vi "HP53220 Measure Frequency w Waveform.vi"(0 "Channel(1,2,3)":enum16{"Channel 1", "Channel 2", "Channel 3"}(ring), 1 "Gate Time":dbl=1.0 min=0.0 max=1000.0 step=0.1 format="%.2f", 5 "Number of Readings":i32=1 min=1, 7 "GPIB Bus":i32 min=0 max=5, 9 "GPIB Address":i16=3 max=31, 11 "error in":errorcluster) -> (2 "Symmetry":dbl format="%.6f", 3 "Frequency":dbl format="%.6f", 4 "Vmax":dbl format="%.6f", 6 "Vmin":dbl format="%.6f", 8 "RTime":dbl format="%.6f", 10 "FTime":dbl format="%.6f", 15 "error out":errorcluster)   [LabVIEW 2023]
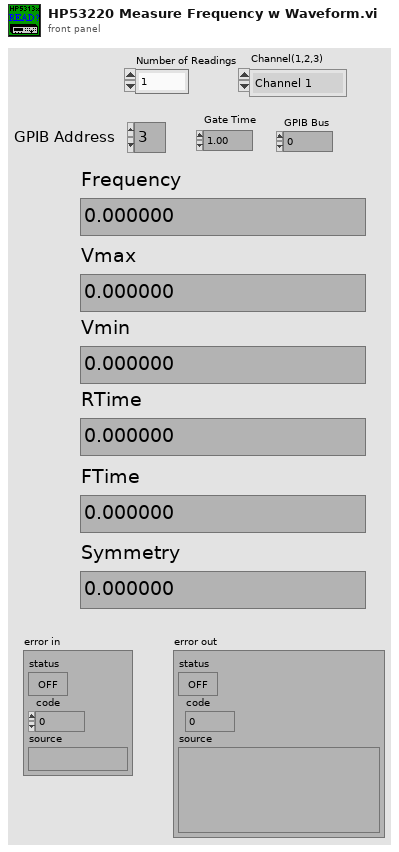
[diagram p1: front panel]
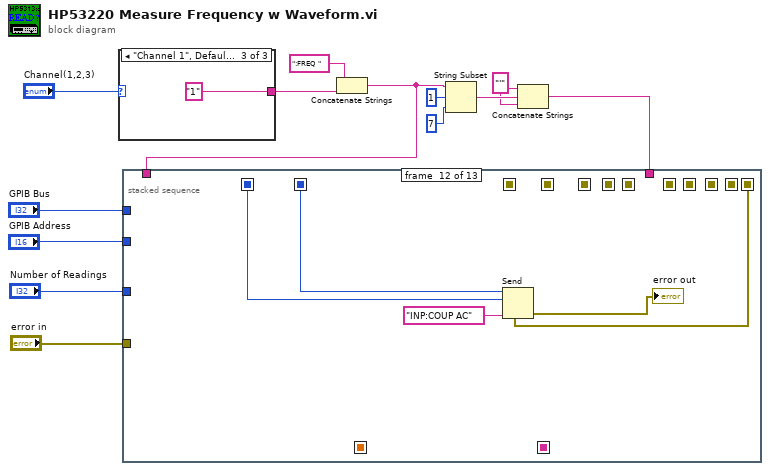
[diagram p0: block diagram]
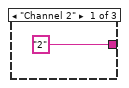
[diagram p2: hidden frame]
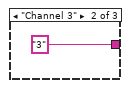
[diagram p3: hidden frame]
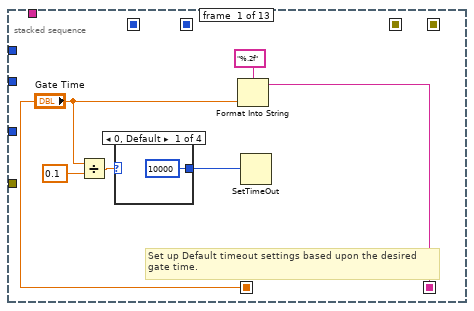
[diagram p4: hidden frame]
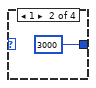
[diagram p5: hidden frame]
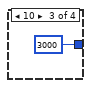
[diagram p6: hidden frame]
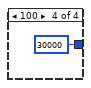
[diagram p7: hidden frame]
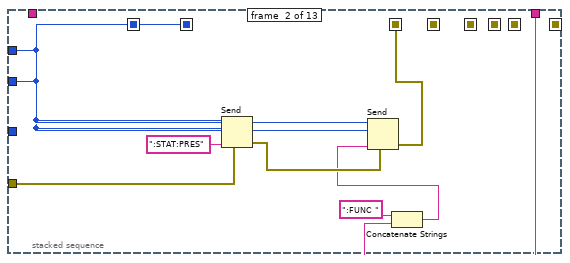
[diagram p8: hidden frame]
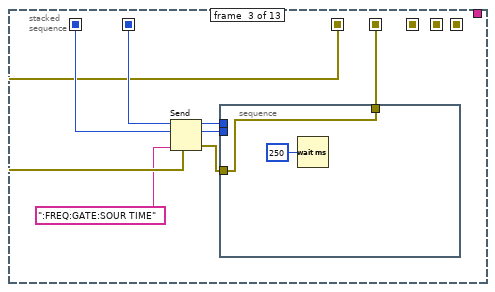
[diagram p9: hidden frame]
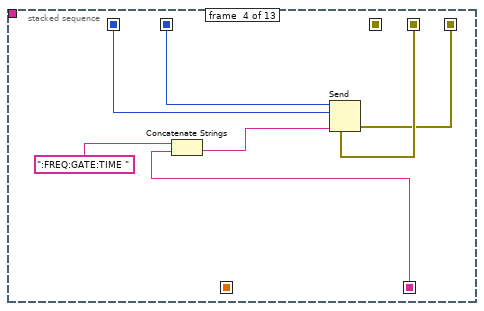
[diagram p10: hidden frame]
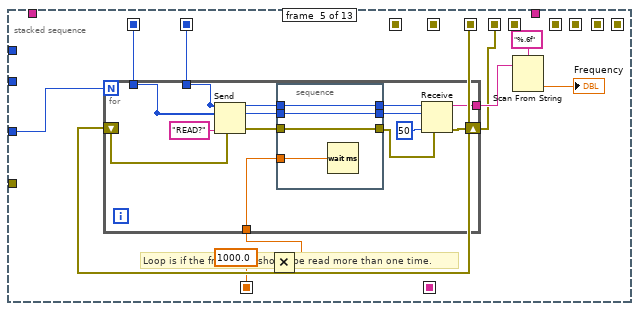
[diagram p11: hidden frame]
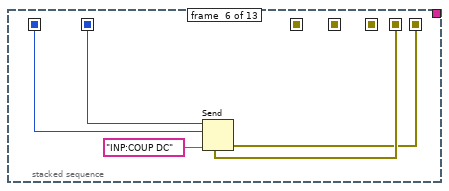
[diagram p12: hidden frame]
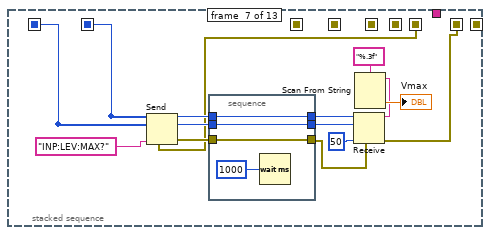
[diagram p13: hidden frame]
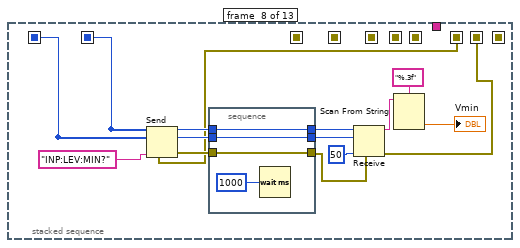
[diagram p14: hidden frame]
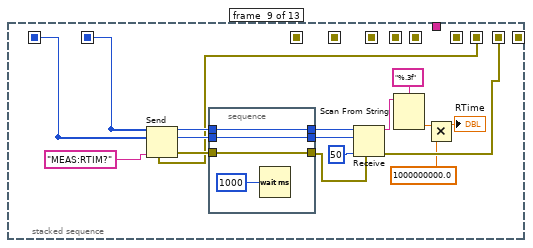
[diagram p15: hidden frame]
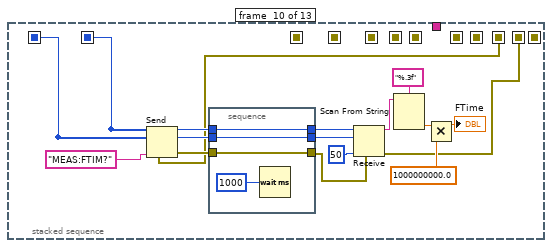
[diagram p16: hidden frame]
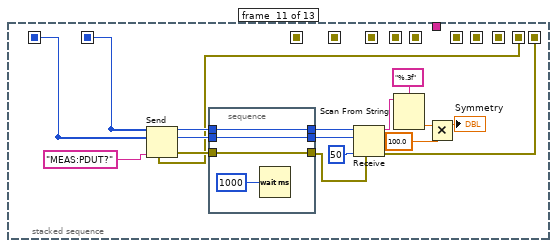
[diagram p17: hidden frame]
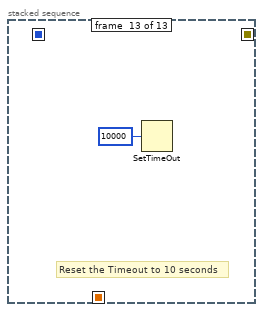
[diagram p18: hidden frame]
diagram:
  w4 = "'"
  n1 = case shown="\"Channel 1\", Default" "Channel(1,2,3)" {
    tunnel: ["2" "3" "1"] -> w10
    frame "Channel 2" {
    }
    frame "Channel 3" {
    }
    frame "Channel 1", Default {
    }
  }
  n2 = Concatenate Strings(":FREQ ", w10) -> (w8:string)
  n3 = String Subset(string=w8, offset (0)=1, length (rest)=7 ("length (rest)")) -> (substring=w5:string)
  n4 = Concatenate Strings(w4, w5, w4) -> (w3:string)
  n5 = stacked-sequence {
    seq-local: [_ w28 _ _ _ _ _ _ _ _ _ _ _] -> [_ _ w40 w50 w55 w81 w89 w106 w125 w144 w163 w177 _]
    seq-local: [w21 _ _ _ _ _ _ _ _ _ _ _ _] -> [_ _ _ w48 _ _ _ _ _ _ _ _ _]
    seq-local: [_ w29 _ _ _ _ _ _ _ _ _ _ _] -> [_ _ w41 w47 w56 w82 w90 w107 w126 w145 w164 w176 _]
    seq-local: [_ w34 _ _ _ _ _ _ _ _ _ _ _] -> [_ _ w39 _ _ _ _ _ _ _ _ _ _]
    seq-local: [_ _ w37 _ _ _ _ _ _ _ _ _ _] -> [_ _ _ w46 _ _ _ _ _ _ _ _ _]
    seq-local: [_ _ _ w45 _ _ _ _ _ _ _ _ _] -> [_ _ _ _ w58 _ _ _ _ _ _ _ _]
    seq-local: ["Gate Time" _ _ _ _ _ _ _ _ _ _ _ _] -> [_ _ _ _ w54 _ _ _ _ _ _ _ _]
    seq-local: [_ _ _ _ w51 _ _ _ _ _ _ _ _] -> [_ _ _ _ _ w79 _ _ _ _ _ _ _]
    seq-local: [_ _ _ _ _ w78 _ _ _ _ _ _ _] -> [_ _ _ _ _ _ w88 _ _ _ _ _ _]
    seq-local: [_ _ _ _ _ _ w83 _ _ _ _ _ _] -> [_ _ _ _ _ _ _ w101 _ _ _ _ _]
    seq-local: [_ _ _ _ _ _ _ w100 _ _ _ _ _] -> [_ _ _ _ _ _ _ _ w121 _ _ _ _]
    seq-local: [_ _ _ _ _ _ _ _ w120 _ _ _ _] -> [_ _ _ _ _ _ _ _ _ w137 _ _ _]
    seq-local: [_ _ _ _ _ _ _ _ _ w136 _ _ _] -> [_ _ _ _ _ _ _ _ _ _ w159 _ _]
    seq-local: [_ _ _ _ _ _ _ _ _ _ w158 _ _] -> [_ _ _ _ _ _ _ _ _ _ _ w175 _]
    tunnel: "GPIB Address" -> [_ w28 _ _ _ _ _ _ _ _ _ _ _]
    tunnel: "GPIB Bus" -> [_ w29 _ _ _ _ _ _ _ _ _ _ _]
    tunnel: w8 -> [_ _ _ _ _ _ _ _ _ _ _ _ _]
    tunnel: w3 -> [_ w30 _ _ _ _ _ _ _ _ _ _ _]
    tunnel: "error in" -> [_ w27 _ _ _ _ _ _ _ _ _ _ _]
    tunnel: "Number of Readings" -> [_ _ _ _ w57 _ _ _ _ _ _ _ _]
    frame #0 {
      # "Set up Default timeout settings based upon the desired \ngate time."
      n6 = Divide(x="Gate Time", y=0.1) -> (x/y=w19:dbl)
      n7 = case shown="0, Default" w19 {
        tunnel: [10000 3000 3000 30000] -> w20
        frame 0, Default {
        }
        frame 1 {
        }
        frame 10 {
        }
        frame 100 {
        }
      }
      n8 = Format Into String(format string="%.2f" ("Format String"), "Gate Time") -> (resulting string=w21:string)  [unwired: 2 in, 1 out]
      n9 = SetTimeOut(1:w20) -> ()  [unwired: 1 out]
    }
    frame #1 {
      n10 = Send(0:w29, 2:w28, 4:w27, 5:":STAT:PRES" ("data string")) -> (8:w33:errorcluster)  [unwired: 1 in, 2 out]
      n11 = Concatenate Strings(":FUNC " ("data string"), w30) -> (w31:string)
      n12 = Send(0:w29, 2:w28, 4:w33, 5:w31) -> (8:w34:errorcluster)  [unwired: 1 in, 2 out]
    }
    frame #2 {
      n13 = Send(0:w41, 2:w40, 4:w39, 5:":FREQ:GATE:SOUR TIME" ("data string")) -> (8:w38:errorcluster)  [unwired: 1 in, 2 out]
      n14 = stacked-sequence {
        tunnel: w41 -> [_]
        tunnel: w40 -> [_]
        tunnel: w38 -> [w42]
        tunnel: [w42] -> w37
        frame #0 {
          n15 = Wait (ms)(milliseconds to wait=u32 250) -> ()  [unwired: 1 out]
        }
      }
    }
    frame #3 {
      n16 = Concatenate Strings(":FREQ:GATE:TIME " ("data string"), w48) -> (w49:string)
      n17 = Send(0:w47, 2:w50, 4:w46, 5:w49) -> (8:w45:errorcluster)  [unwired: 1 in, 2 out]
    }
    frame #4 {
      # "Loop is if the frequency should be read more than one time."
      n18 = Multiply(x=1000.0, y=w54) -> (x*y=w52:dbl)
      n19 = for {
        N: w57 -> [_]
        tunnel: w55 -> [w64]
        tunnel: w56 -> [w63]
        tunnel: [w72] -> w59
        shift-right: [w69] -> w51
        shift-left: w58 -> [w71]
        tunnel: w52 -> [w68]
        n20 = Send(0:w63, 2:w64, 4:w71, 5:"READ?" ("data string")) -> (8:w67:errorcluster)  [unwired: 1 in, 2 out]
        n21 = stacked-sequence {
          tunnel: w68 -> [w77]
          tunnel: w67 -> [w74]
          tunnel: [w75] -> w66
          tunnel: [w76] -> w65
          tunnel: w64 -> [w76]
          tunnel: w63 -> [w75]
          tunnel: [w74] -> w62
          frame #0 {
            n22 = Wait (ms)(milliseconds to wait=w77) -> ()  [unwired: 1 out]
          }
        }
        n23 = Receive(4:w62, 6:50 ("count"), 8:w65, 9:w66) -> (0:w69:errorcluster, 3:w72:string)  [unwired: 1 in, 2 out]
      }
      n24 = Scan From String(format string="%.6f" ("Format String"), input string=w59) -> (output 1=→"Frequency":dbl)  [unwired: 3 in, 3 out]
    }
    frame #5 {
      n25 = Send(0:w82, 2:w81, 4:w79, 5:"INP:COUP DC" ("data string")) -> (8:w78:errorcluster)  [unwired: 1 in, 2 out]
    }
    frame #6 {
      n26 = Send(0:w90, 2:w89, 4:w88, 5:"INP:LEV:MAX?" ("data string")) -> (8:w94:errorcluster)  [unwired: 1 in, 2 out]
      n27 = stacked-sequence {
        tunnel: w94 -> [w97]
        tunnel: [w98] -> w93
        tunnel: [w99] -> w92
        tunnel: w89 -> [w99]
        tunnel: w90 -> [w98]
        tunnel: [w97] -> w91
        frame #0 {
          n28 = Wait (ms)(milliseconds to wait=u32 1000) -> ()  [unwired: 1 out]
        }
      }
      n29 = Receive(4:w91, 6:50 ("count"), 8:w92, 9:w93) -> (0:w83:errorcluster, 3:w86:string)  [unwired: 1 in, 2 out]
      n30 = Scan From String(format string="%.3f" ("Format String"), input string=w86) -> (output 1=→"Vmax":dbl)  [unwired: 3 in, 3 out]
    }
    frame #7 {
      n31 = Send(0:w107, 2:w106, 4:w101, 5:"INP:LEV:MIN?" ("data string")) -> (8:w111:errorcluster)  [unwired: 1 in, 2 out]
      n32 = stacked-sequence {
        tunnel: w111 -> [w114]
        tunnel: [w115] -> w110
        tunnel: [w116] -> w109
        tunnel: w106 -> [w116]
        tunnel: w107 -> [w115]
        tunnel: [w114] -> w108
        frame #0 {
          n33 = Wait (ms)(milliseconds to wait=u32 1000) -> ()  [unwired: 1 out]
        }
      }
      n34 = Receive(4:w108, 6:50 ("count"), 8:w109, 9:w110) -> (0:w100:errorcluster, 3:w104:string)  [unwired: 1 in, 2 out]
      n35 = Scan From String(format string="%.3f" ("Format String"), input string=w104) -> (output 1=→"Vmin":dbl)  [unwired: 3 in, 3 out]
    }
    frame #8 {
      n36 = Send(0:w126, 2:w125, 4:w121, 5:"MEAS:RTIM?" ("data string")) -> (8:w130:errorcluster)  [unwired: 1 in, 2 out]
      n37 = stacked-sequence {
        tunnel: w130 -> [w133]
        tunnel: [w134] -> w129
        tunnel: [w135] -> w128
        tunnel: w125 -> [w135]
        tunnel: w126 -> [w134]
        tunnel: [w133] -> w127
        frame #0 {
          n38 = Wait (ms)(milliseconds to wait=u32 1000) -> ()  [unwired: 1 out]
        }
      }
      n39 = Receive(4:w127, 6:50 ("count"), 8:w128, 9:w129) -> (0:w120:errorcluster, 3:w124:string)  [unwired: 1 in, 2 out]
      n40 = Scan From String(format string="%.3f" ("Format String"), input string=w124) -> (output 1=w119:dbl)  [unwired: 3 in, 3 out]
      n41 = Multiply(x=w119, y=1000000000.0) -> (x*y=→"RTime":dbl)
    }
    frame #9 {
      n42 = Send(0:w145, 2:w144, 4:w137, 5:"MEAS:FTIM?" ("data string")) -> (8:w149:errorcluster)  [unwired: 1 in, 2 out]
      n43 = stacked-sequence {
        tunnel: w149 -> [w152]
        tunnel: [w153] -> w148
        tunnel: [w154] -> w147
        tunnel: w144 -> [w154]
        tunnel: w145 -> [w153]
        tunnel: [w152] -> w146
        frame #0 {
          n44 = Wait (ms)(milliseconds to wait=u32 1000) -> ()  [unwired: 1 out]
        }
      }
      n45 = Receive(4:w146, 6:50 ("count"), 8:w147, 9:w148) -> (0:w136:errorcluster, 3:w143:string)  [unwired: 1 in, 2 out]
      n46 = Scan From String(format string="%.3f" ("Format String"), input string=w143) -> (output 1=w140:dbl)  [unwired: 3 in, 3 out]
      n47 = Multiply(x=w140, y=1000000000.0) -> (x*y=→"FTime":dbl)
    }
    frame #10 {
      n48 = Send(0:w164, 2:w163, 4:w159, 5:"MEAS:PDUT?" ("data string")) -> (8:w168:errorcluster)  [unwired: 1 in, 2 out]
      n49 = stacked-sequence {
        tunnel: w168 -> [w171]
        tunnel: [w172] -> w167
        tunnel: [w173] -> w166
        tunnel: w163 -> [w173]
        tunnel: w164 -> [w172]
        tunnel: [w171] -> w165
        frame #0 {
          n50 = Wait (ms)(milliseconds to wait=u32 1000) -> ()  [unwired: 1 out]
        }
      }
      n51 = Receive(4:w165, 6:50 ("count"), 8:w166, 9:w167) -> (0:w158:errorcluster, 3:w162:string)  [unwired: 1 in, 2 out]
      n52 = Scan From String(format string="%.3f" ("Format String"), input string=w162) -> (output 1=w157:dbl)  [unwired: 3 in, 3 out]
      n53 = Multiply(x=w157, y=100.0) -> (x*y=→"Symmetry":dbl)
    }
    frame #11 {
      n54 = Send(0:w176, 2:w177, 4:w175, 5:"INP:COUP AC" ("data string")) -> (8:→"error out":errorcluster)  [unwired: 1 in, 2 out]
    }
    frame #12 {
      # "Reset the Timeout to 10 seconds"
      n55 = SetTimeOut(1:10000 ("new timeout (10000)")) -> ()  [unwired: 1 out]
    }
  }
